vi "VI_1.vi"(8 "error in (no error)":errorcluster, 11 "Ports in":refnum<class "Ports.lvclass">) -> (0 "error out":errorcluster, 3 "Ports out":refnum<class "Ports.lvclass">)   [LabVIEW 2010, in "Ports.lvclass"]
uses:
  Ports.lvclass
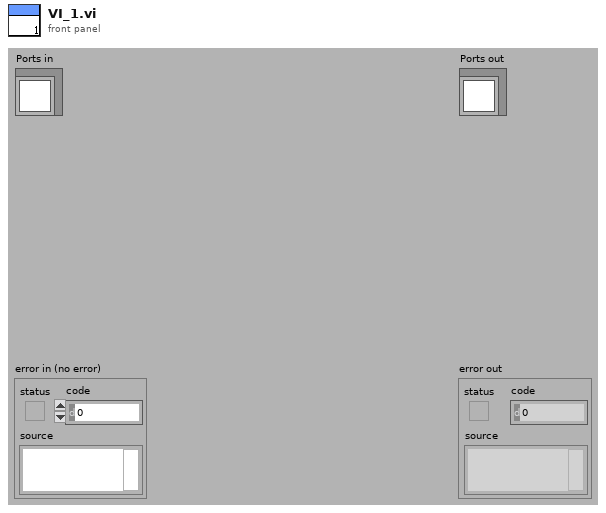
[diagram p1: front panel]
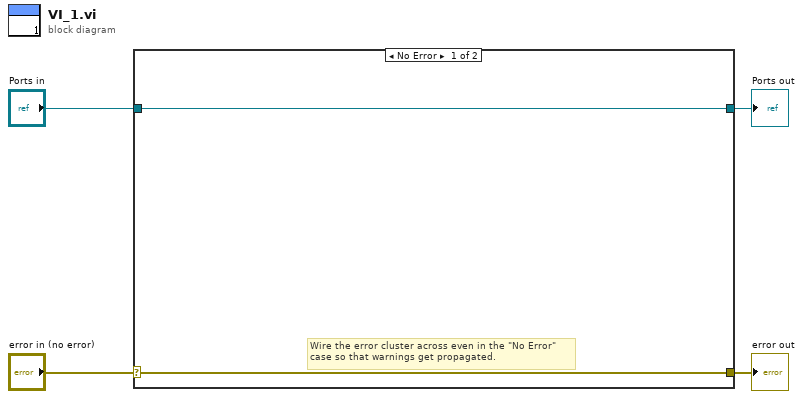
[diagram p0: block diagram]
diagram:
  n1 = case shown="No Error" "error in (no error)" {
    selector: "error in (no error)" -> [w5 w8]
    tunnel: [w5 w8] -> w3
    tunnel: [w6 w7] -> w1
    tunnel: "Ports in" -> [w6 w7]
    frame No Error {
      # "Wire the error cluster across even in the \"No Error\"\ncase so that warnings get propagated."
    }
    frame Error {
    }
  }
  "error out" <- w3
  "Ports out" <- w1
